vi "tb_test fifo full.vi"(9 "fifo depth":u8(ring)=10 items=["4"=2, "8"=3, "16"=4, "32"=5, "64"=6, "128"=7, "256"=8, "512"=9, "1024"=10, "2048"=11, "4096"=12, "8192"=13, "16384"=14, "32768"=15, "65536"=16, "131072"=17, "262144"=18, "524288"=19, "1048576"=20, "2097152"=21, "4194304"=22, "8388608"=23, "16777216"=24, "33554432"=25, "67108864"=26, "134217728"=27, "268435456"=28, "536870912"=29, "1073741824"=30, "2147483648"=31, "4294967296"=32], 10 "arbiter configuration":T1={"write grant time (clocks)"=100, "read grant time (clocks)"=100}, 11 "Memory":T2={"fifo1 memory"="Bank0", "fifo2 memory"="Bank1"}) -> (3 "Pass?":bool=TRUE)   [LabVIEW 2011]
uses:
  <instrlib>/RF-RIO/Memory/FPGA/Interface/Timeslot Arbiter Configuration.ctl
  Data Type (256).ctl
  <instrlib>/RF-RIO/Memory/FPGA/Memory.lvlib
panel:
  out "FIFO Full":bool[](array[boolean])
  out "Ready for Input":bool[](array[boolean])
  out "Iteration":i32
  # "1) Set Ready for Output\n2) Input FIFO Size + Maximum Outstanding Read Requests\n3) Check if the is FIFO Full Status goes high at the end of test bench \n4) Check if Ready for Input goes low when FIFO Full Status is high\n3 & 4 Pass=> Test Passed"
  # "Debug Area"
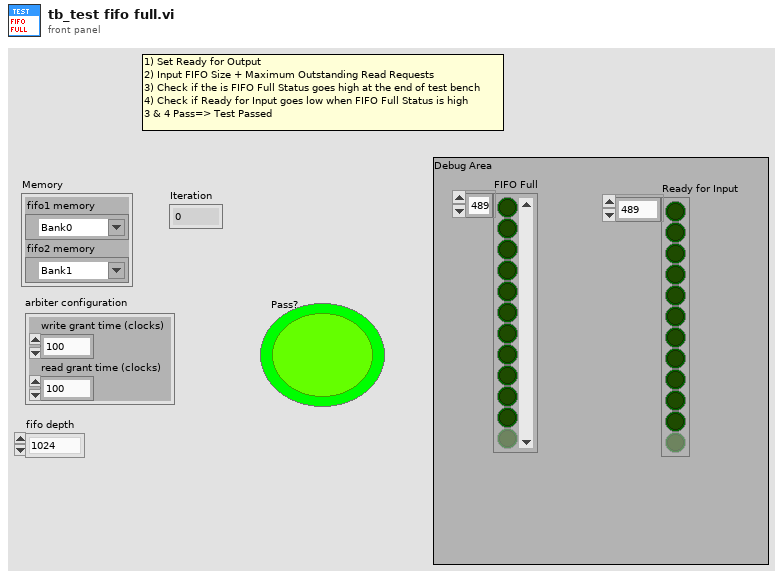
[diagram p1: front panel]
types:
  T1 = typedef "Memory.lvlib/Timeslot Arbiter Configuration.ctl" = cluster{"write grant time (clocks)":u16, "read grant time (clocks)":u16}
  T2 = cluster{"fifo1 memory":refnum<k21>, "fifo2 memory":refnum<k21>}
  T3 = typedef "Data Type (256).ctl" = cluster{"Bank0. High":u64, "Bank0. Low":u64, "Bank1. High":u64, "Bank1. Low":u64}
  T4 = typedef "FIFO.lvlib/FIFO State.ctl" = cluster{"write address":u32, "read address":u32, "full count":u32, "full":bool, "empty":bool, "in reset":bool}
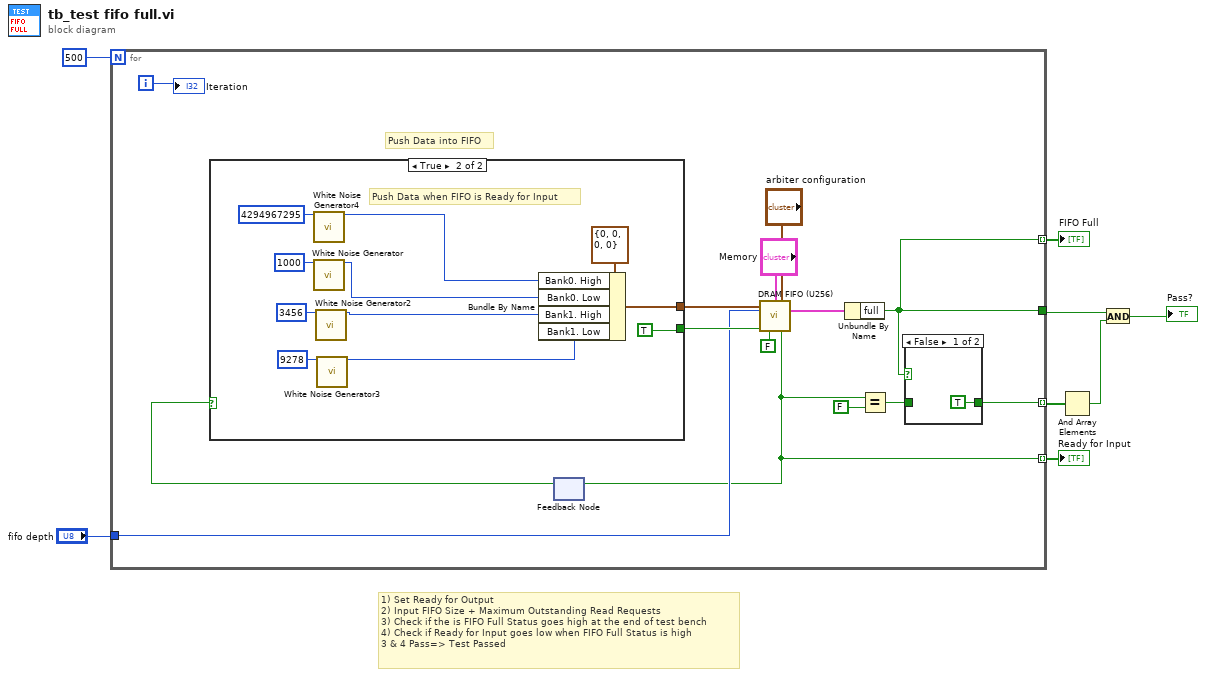
[diagram p0: block diagram]
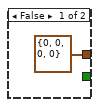
[diagram p3: hidden frame]
diagram:
  # "1) Set Ready for Output\n2) Input FIFO Size + Maximum Outstanding Read Requests\n3) Check if the is FIFO Full Status goes high at the end of test bench \n4) Check if Ready for Input goes low when FIFO Full Status is high\n3 & 4 Pass=> Test Passed"
  n1 = for {
    N: 500 -> [_]
    tunnel: "fifo depth" -> [w16]
    tunnel: [w9] -> w4
    tunnel: [w13] -> w6 mode=indexing
    tunnel: [w10] -> w5 mode=indexing
    tunnel: [w9] -> w1 mode=indexing
    i -> [w18]
    # "Push Data into FIFO"
    n2 = feedback #1() -> (w21:bool)  [unwired: 1 in]
    n3 = case shown="True" w21 {
      tunnel: [T3 {"Bank0. High"=0, "Bank0. Low"=0, "Bank1. High"=0, "Bank1. Low"=0} ("Input Data") w35] -> w20
      tunnel: [_ TRUE] -> w19
      frame False {
      }
      frame True {
        # "Push Data when FIFO is Ready for Input"
        n4 = call "White Noise Generator4"("seed"=u32 4294967295) -> ("white noise out"=w26:i16)  [unwired: 14 in]
        n5 = call "White Noise Generator"("seed"=u32 1000) -> ("white noise out"=w27:i16)  [unwired: 14 in]
        n6 = call "White Noise Generator2"("seed"=u32 3456) -> ("white noise out"=w28:i16)  [unwired: 14 in]
        n7 = call "White Noise Generator3"("seed"=u32 9278) -> ("white noise out"=w29:i16)  [unwired: 14 in]
        n8 = Bundle By Name(cluster=T3 {"Bank0. High"=0, "Bank0. Low"=0, "Bank1. High"=0, "Bank1. Low"=0} ("Input Data"), "Bank0. High"=w26, "Bank0. Low"=w27, "Bank1. High"=w28, "Bank1. Low"=w29) -> (w35:T3)
      }
    }
    n9 = call "DRAM FIFO (U256).vi"("Input Data"=w20, "Memory"="Memory", "arbiter configuration"="arbiter configuration", "fifo depth"=w16, "input valid"=w19, "ready for output"=FALSE) -> ("state"=w14:T4, "Ready for Input"=w13:bool)  [unwired: 4 in, 4 out]
    n10 = feedback-in #1(w13) -> ()
    n11 = Unbundle By Name(w14) -> ("full"=w9:bool)
    n12 = Equal?(x=w13, y=FALSE) -> (x = y?=w11:bool)
    n13 = case shown="False" w9 {
      tunnel: w11 -> [_ w24]
      tunnel: [TRUE w24] -> w10
      frame False {
      }
      frame True {
      }
    }
    "Iteration" <- w18
  }
  "Ready for Input" <- w6
  "FIFO Full" <- w1
  n14 = And Array Elements(Boolean array=w5) -> (logical AND=w3:bool)
  n15 = And(x=w4, y=w3) -> (x .and. y?=→"Pass?":bool)
